vi "HSDIO_6541_Run.vi"(8 "error  in":errorcluster caption="error in", 10 "Use Software trigger":bool, 11 "instrument handle in":refnum<k15>="HSDIO_6541") -> (0 "error out":errorcluster, 3 "instrument handle out":refnum<k15>)   [LabVIEW 2018]
doc: "I Description: FOR TESTS PURPOSE ONLY\nThis VI inits a waveform generation session for HSDIO 6541. This is a basic example that shows how to setup the board in order to generate waveforms according to a script. \n\nII Instructions for Running:\n1. Start the VI and select any previously created sequence script.\n2. If software trigger is choosen, just click on the Send Software Trigger button to generate the sequence.\nIf not, connect an external TTL trigger to the PFI0 input pin of the HSDIO, and generation will start immediately after the next trigger pulse.\n\nIII Block Diagram Steps:\n1. Initialize for a generation session.\n2. Assign the specified channels in Channel List for dynamic operation.\n3. Configure the Sample clock to use the onboard clock, and configure the clock rate.\n\n\n\n1. Initialize for a generation session.\n2. Assign specified channels in Channel List for dynamic operation : all = \"\" (default)\n3. Sets the Idle State for when the generation has completed : NO !!\n4. Configure the Sample clock to use the onboard clock, and configure the clock rate.\n5. Set generation mode to Scripted.\n6. Configure the Script Trigger : change to Digital Edge if waiting for an external\n trigger, and link Rising Edge and source trigger commands.\n Use PFI0 with SMB wired to the board, or any PFIxx if connected to accessory.\n6. Initiate dynamic pattern generation.\n7. Wait until the generation is done.\n8. Close the generation session."
uses:
  <instrlib>/niHSDIO/niHSDIO.llb/niHSDIO_ctl Trigger SW - TrigIdentifier Values (Ring).ctl
  <instrlib>/niHSDIO/niHSDIO.llb/niHSDIO_ctl Trigger SW - TrigName Values (Ring).ctl
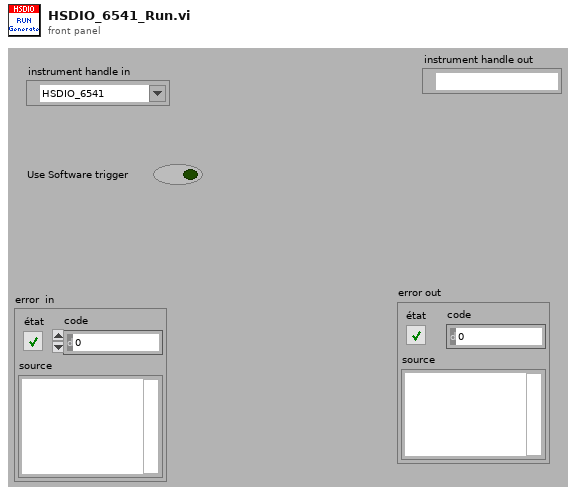
[diagram p1: front panel]
types:
  T1 = typedef "niHSDIO_ctl Trigger SW - TrigIdentifier Values (Ring).ctl" = string
  T2 = typedef "niHSDIO_ctl Trigger SW - TrigName Values (Ring).ctl" = i32
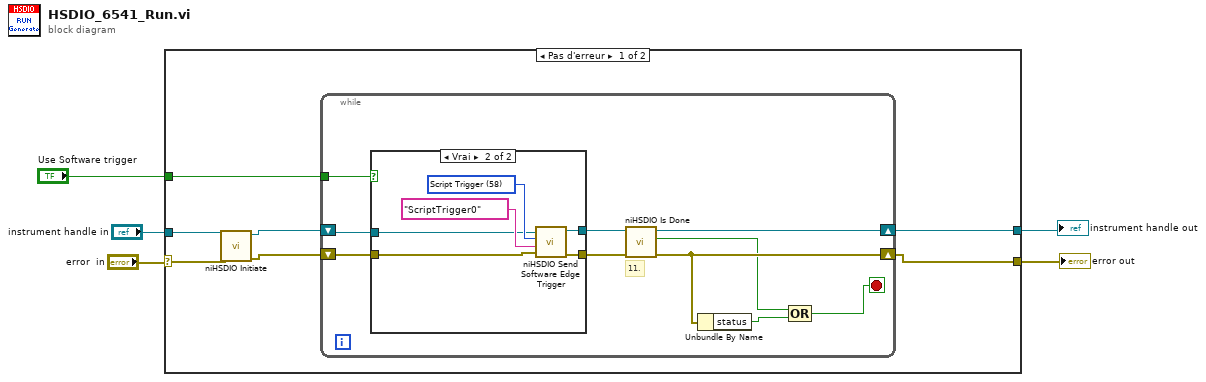
[diagram p0: block diagram]
diagram:
  n1 = case shown="Pas d'erreur" "error  in" {
    selector: "error  in" -> [w9 w31]
    tunnel: "instrument handle in" -> [w11 w32]
    tunnel: [w7 w32] -> w4
    tunnel: [w6 w31] -> w3
    tunnel: "Use Software trigger" -> [w12 _]
    frame No Error {
      n2 = call <instrlib>:"niHSDIO Initiate.vi"("error in (no error)"=w9, "instrument handle"=w11) -> ("error out"=w8:errorcluster, "instrument handle out"=w10:refnum<k15>)  [unwired: 8 in]
      n3 = while {
        tunnel: w12 -> [w18]
        shift-right: [w19] -> w7
        shift-left: w10 -> [w21]
        shift-right: [w16] -> w6
        shift-left: w8 -> [w22]
        stop <- w13 stop-if-true
        # "11."
        n4 = case shown="Vrai" w18 {
          tunnel: [w23 w30] -> w20
          tunnel: [w24 w29] -> w17
          tunnel: w22 -> [w24 w26]
          tunnel: w21 -> [w23 w25]
          frame False {
          }
          frame True {
            w27 = T2 58 items=["Start Trigger"=53, "Reference Trigger"=54, "Advance Trigger"=61, "Script Trigger"=58, "Stop Trigger"=82] ("trigger (start trigger)")
            n5 = call <instrlib>:"niHSDIO Send Software Edge Trigger.vi"("error in (no error)"=w26, "trigger identifier (none)"=T1 "ScriptTrigger0", "trigger (start trigger)"=w27, "instrument handle"=w25) -> ("error out"=w29:errorcluster, "instrument handle out"=w30:refnum<k15>)  [unwired: 6 in]
          }
        }
        n6 = call <instrlib>:"niHSDIO Is Done.vi"("error in (no error)"=w17, "instrument handle"=w20) -> ("error out"=w16:errorcluster, "done"=w15:bool, "instrument handle out"=w19:refnum<k15>)  [unwired: 7 in]
        n7 = Unbundle By Name(w16) -> ("status"=w14:bool)
        n8 = Compound Arithmetic op=OR ("Opérateur arithmétique")(w15, w14) -> (w13:bool)
      }
    }
    frame Error {
    }
  }
  "error out" <- w3
  "instrument handle out" <- w4
